vi "Refresh Stats.vi"(7 "Plugin Name":string, 8 "error in (no error)":errorcluster, 10 "Index":i32, 11 "CIF_Plugin_UI in":refnum<class "CIF_UI.lvclass">) -> (0 "error out":errorcluster, 1 "Not Found":bool, 3 "CIF_Plugin_UI out":refnum<class "CIF_UI.lvclass">)   [LabVIEW 2021, in "CIF_UI.lvclass"]
uses:
  CIF_UI.lvclass
  CIFCore/Grpc/CIFCoreWrapper/CIFCoreWrapper.lvlib
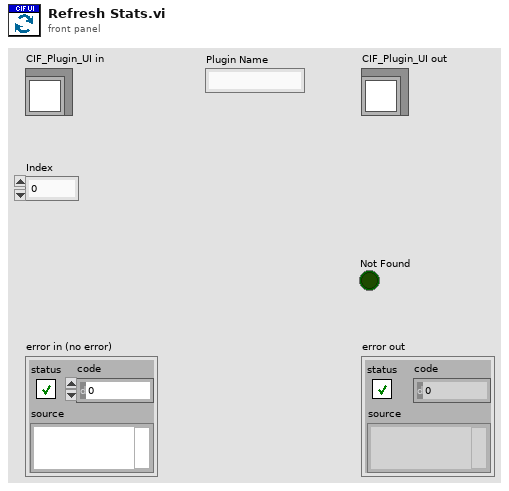
[diagram p1: front panel]
types:
  T1 = typedef "grpc-lvsupport-release.lvlib/grpcId.ctl" = u64
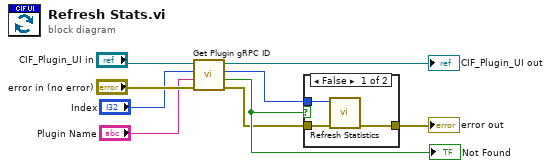
[diagram p0: block diagram]
diagram:
  n1 = call "Get Plugin gRPC ID.vi"("error in (no error)"="error in (no error)", "Plugin Name"="Plugin Name", "Index"="Index", "CIF_UI in"="CIF_Plugin_UI in") -> ("error out"=w3:errorcluster, "Not Found"=w4:bool, "gRPC ID"=w5:T1, "CIF_UI out"=→"CIF_Plugin_UI out":refnum<class "CIF_UI.lvclass">)  [unwired: 3 in, 1 out]
  "Not Found" <- w4
  n2 = case shown="False" w4 {
    tunnel: w5 -> [w12 _]
    tunnel: w3 -> [w11 w13]
    tunnel: [w10 w13] -> w2
    frame False {
      n3 = call "Refresh Statistics.vi"("error in"=w11, "gRPC ID"=w12) -> ("error out"=w10:errorcluster)  [unwired: 8 in, 1 out]
    }
    frame True {
    }
  }
  "error out" <- w2
